vi "ADIS16448_RoboRIO_Teensy_GetData.vi"(8 "error in":errorcluster, 11 "SerialPortRefIn":T2) -> (0 "error out":errorcluster, 1 "IMU AHRS Out":cluster{"Pitch":dbl, "Roll":dbl, "Yaw":dbl}, 2 "IMU Angles Out":T1, 3 "SerialPortRefOut":T2)   [LabVIEW 2016, in "RoboRIO-Teensy-ADIS16448-Interface.lvlib"]
uses:
  RoboRIO-Teensy-ADIS16448-Interface.lvlib
  <vilib>/Rock Robotics/WPI/SerialPort/WPI_SerialPortRef.ctl
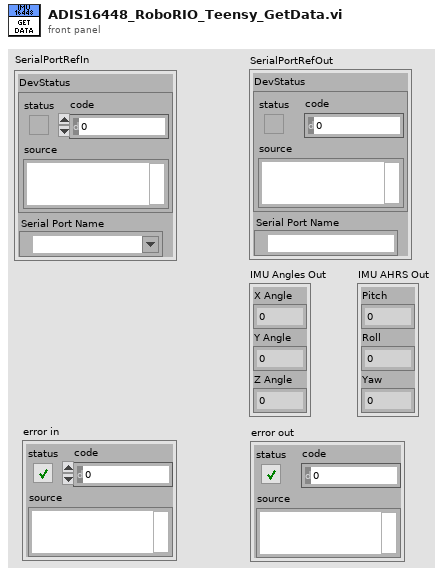
[diagram p1: front panel]
types:
  T1 = cluster{"X Angle":dbl, "Y Angle":dbl, "Z Angle":dbl}
  T2 = typedef "WPI_SerialPortRef.ctl" = cluster{"DevStatus":errorcluster, "Serial Port Name":refnum<visa-resource-name>}
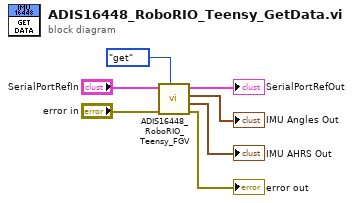
[diagram p0: block diagram]
diagram:
  n1 = call "ADIS16448_RoboRIO_Teensy_FGV.vi"("Operation"=enum16{"set", "get", "set reset"}."get", "error in"="error in", "SerialPortRefIn"="SerialPortRefIn") -> ("error out"=→"error out":errorcluster, "IMU AHRS Out"=→"IMU AHRS Out":cluster{"Pitch":dbl, "Roll":dbl, "Yaw":dbl}, "IMU Angles Out"=→"IMU Angles Out":T1, "SerialPortRefOut"=→"SerialPortRefOut":T2)  [unwired: 4 in, 1 out]
